vi "给表格某列赋值.vi"(8 "错误输入（无错误）":errorcluster, 9 "列数":i32, 10 "内容":string[](array[string]), 11 "引用输入":refnum<vi>) -> (0 "错误输出":errorcluster, 3 "引用输出":refnum<vi>)   [LabVIEW 2014, in "表格.lvlib"]
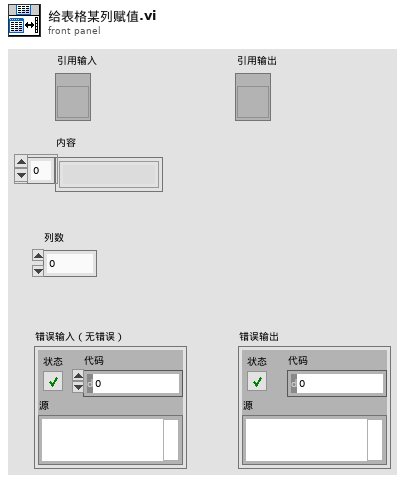
[diagram p1: front panel]
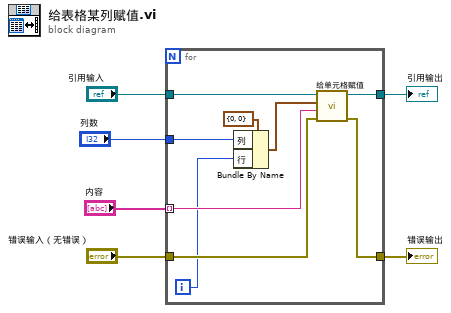
[diagram p0: block diagram]
diagram:
  n1 = for {
    tunnel: "引用输入" -> [w15]
    tunnel: [w14] -> w5
    tunnel: "错误输入（无错误）" -> [w13]
    tunnel: [w12] -> w3
    tunnel: "内容" -> [w11] mode=indexing
    tunnel: "列数" -> [w8]
    i -> [w7]
    n2 = Bundle By Name(cluster=cluster{"行":i32, "列":i32} {"行"=0, "列"=0} ("行列"), "列"=w8, "行"=w7) -> (w9:cluster{"行":i32, "列":i32})
    n3 = call "给单元格赋值.vi"("错误输入（无错误）"=w13, "新元素/子数组"=w11, "行列"=w9, "引用输入"=w15) -> ("错误输出"=w12:errorcluster, "引用输出"=w14:refnum<vi>)  [unwired: 6 in]
  }
  "引用输出" <- w5
  "错误输出" <- w3
